vi "AMC Read Next Message.vi"(8 "error in (no error)":errorcluster, 9 "Termination List ([Exit])":string[](array[string])=["Exit"], 10 "timeout (1ms)":i32=1, 11 "Message Queue in":T3) -> (0 "error out":errorcluster, 1 "Message Value":string, 2 "Message Name":string, 3 "Message Queue out":T3, 4 "Message Attributes":T1, 5 "Exit Process":bool, 6 "Message":T2)   [LabVIEW 2009]
doc: "This VI is used for compatibility with previous versions of the AMC library. Use the AMC VIs located in the <b>Data Communication >> Asynchronous Message Communication</b> palette."
uses:
  Message Queue.ctl
  Message.ctl
  <vilib>/NI/Tools/Keyed Array/KeyedArray.ctl
  AMC.lvlib
  <vilib>/NI/Tools/Keyed Array/Tools_KeyedArray.lvlib
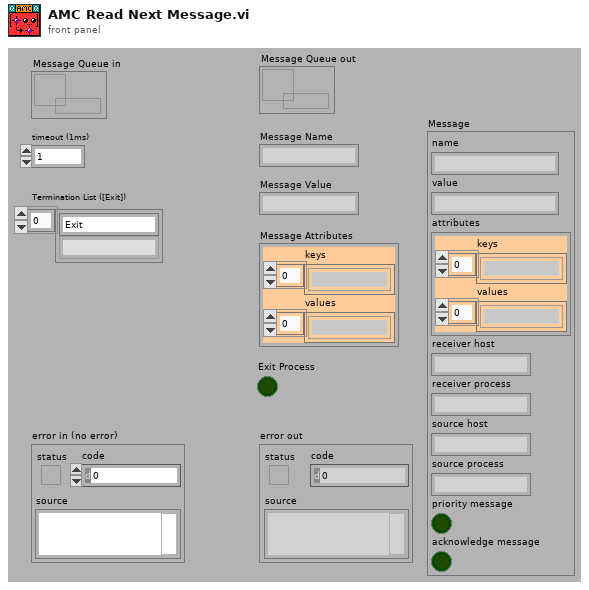
[diagram p1: front panel]
types:
  T1 = typedef "Tools_KeyedArray.lvlib/KeyedArray.ctl" = cluster{"keys":string[], "values":string[]}
  T2 = typedef "AMC.lvlib/Message.ctl" = cluster{"name":string, "value":string, "attributes":T1, "receiver host":string, "receiver process":string, "source host":string, "source process":string, "priority message":bool, "acknowledge message":bool}
  T3 = typedef "AMC.lvlib/Message Queue.ctl" = refnum<queue>
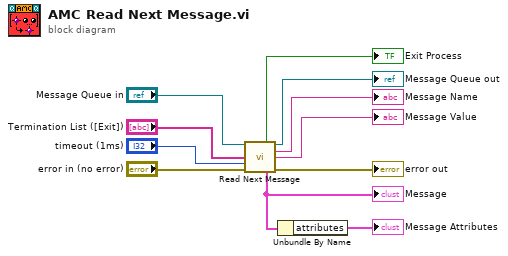
[diagram p0: block diagram]
diagram:
  n1 = call "Read Next Message.vi"("message queue in"="Message Queue in", "termination list ([Exit])"="Termination List ([Exit])", "timeout (1 ms)"="timeout (1ms)", "error in"="error in (no error)") -> ("exit process?"=→"Exit Process":bool, "message queue out"=→"Message Queue out":T3, "message name"=→"Message Name":string, "message value"=→"Message Value":string, "message"=w2:T2, "error out"=→"error out":errorcluster)  [unwired: 4 in, 2 out]
  "Message" <- w2
  n2 = Unbundle By Name(w2) -> ("attributes"=→"Message Attributes":T1)
